vi "setPollerPath.vi"(8 "error in (no error)":errorcluster, 10 "pollerPath":string, 11 "ttm_poller_panel.vi in":refnum<class "ttm_poller_panel.vi.lvclass">) -> (0 "error out":errorcluster, 3 "ttm_poller_panel.vi out":refnum<class "ttm_poller_panel.vi.lvclass">)   [LabVIEW 2009, in "ttm_poller_panel.vi.lvclass"]
uses:
  ttm_poller_panel.vi.lvclass
  ttm_poller_panel.vi.lvclass/ttm_poller_panel.vi.ctl
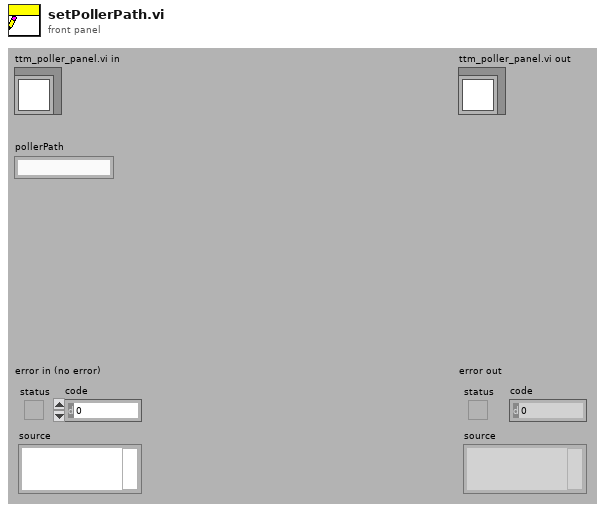
[diagram p1: front panel]
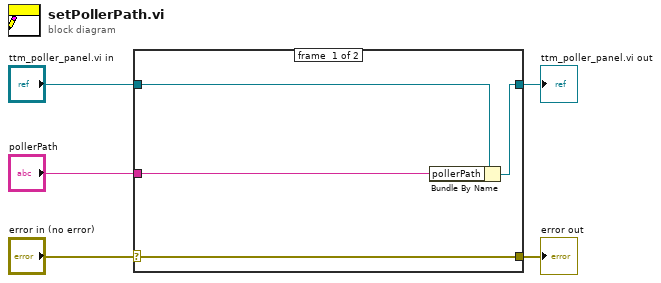
[diagram p0: block diagram]
diagram:
  n1 = case shown="No Error" "error in (no error)" {
    selector: "error in (no error)" -> [w9 w10]
    tunnel: [w9 w10] -> w4
    tunnel: [w7 w11] -> w2
    tunnel: "ttm_poller_panel.vi in" -> [w8 w11]
    tunnel: "pollerPath" -> [w6 _]
    frame #0 {
      n2 = Bundle By Name(cluster=w8, "pollerPath"=w6) -> (w7:refnum<class "ttm_poller_panel.vi.lvclass">)
    }
    frame #1 {
    }
  }
  "error out" <- w4
  "ttm_poller_panel.vi out" <- w2
